vi "Renishaw-XL80_SetFastAveraging.vi"(8 "error in (no error)":errorcluster, 11 "Renishaw-XL80_EMU in":refnum<class "Renishaw-XL80_EMU.lvclass">) -> (0 "error out":errorcluster, 3 "Renishaw-XL80_EMU out":refnum<class "Renishaw-XL80_EMU.lvclass">)   [LabVIEW 2024, in "Renishaw-XL80_EMU.lvclass"]
doc: "This method will set short-term averaging of the ML10 reading on.\n\nDefinition\nHRESULTSetSlowAveraging();\nParameters\nNone\n\nComments\nThis method will return with an HRESULT of E_FAIL if the client has not previously connected to a DX10 by calling Connect. The method will also return E_FAIL if the DX10 is not responding or the ML10 is not responding. Otherwise the method will return an HRESULT of S_OK.\n\nShort term (fast) averaging enables a \"box car\" averaging algorithm inside the ML10 with a response time of approximately 1/4sec.\n\nNote that short term averaging is on when the ML10 status has ML10_AVERAGING_ON set and ML10_LONG_TERM_AVERAGING_ON not set.\n\nNote that averaging has no effect on synchronous TPin triggered readings."
uses:
  Renishaw-XL80_EMU.lvclass
  Renishaw-XL80_EMU.lvclass/Renishaw-XL80_EMU.ctl
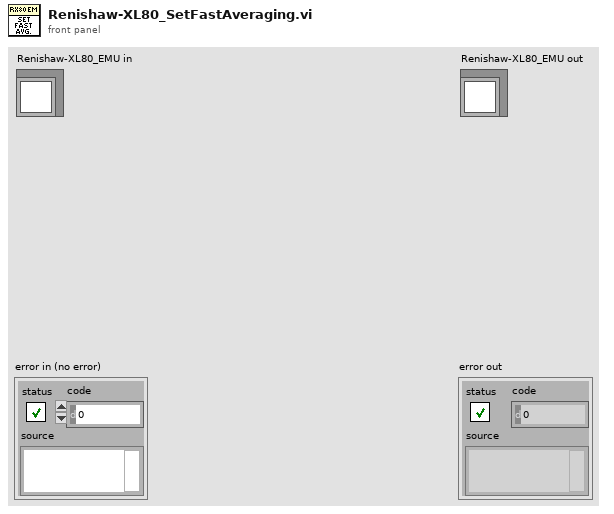
[diagram p1: front panel]
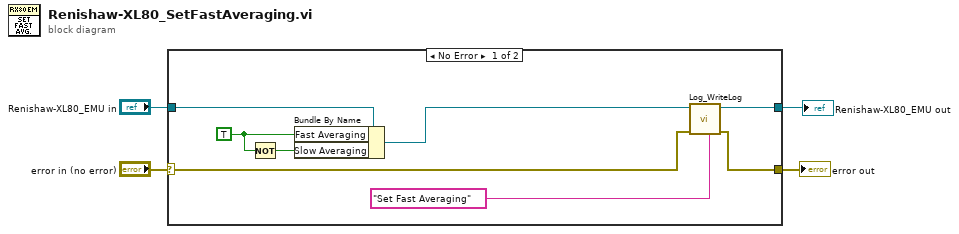
[diagram p0: block diagram]
diagram:
  n1 = case shown="No Error" "error in (no error)" {
    selector: "error in (no error)" -> [w9 w13]
    tunnel: [w10 w14] -> w1
    tunnel: "Renishaw-XL80_EMU in" -> [w12 w14]
    tunnel: [w8 w13] -> w2
    frame No Error {
      w6 = TRUE ("Fast Averaging")
      n2 = Not(x=w6) -> (.not. x?=w5:bool)
      n3 = Bundle By Name(cluster=w12, "Fast Averaging"=w6, "Slow Averaging"=w5) -> (w11:refnum<class "Renishaw-XL80_EMU.lvclass">)
      n4 = call-dynamic "Log_WriteLog.vi"("Additional text"="Set Fast Averaging", "error in (no error)"=w9, "Log in"=w11) -> ("error out"=w8:errorcluster, "Log out"=w10:refnum<class "Renishaw-XL80_EMU.lvclass">)  [unwired: 7 in]
    }
    frame Error {
    }
  }
  "error out" <- w2
  "Renishaw-XL80_EMU out" <- w1
